vi "Pre Launch Init.vi"(11 "Topic in":refnum<class "Topic.lvclass">) -> (0 "error out":errorcluster, 3 "Topic out":refnum<class "Topic.lvclass">)   [LabVIEW 2017, in "Mediator.lvlib" / "Topic.lvclass"]
doc: "(<B>Filename</B>: Actor Framework.lvlib:Actor.lvclass:Pre Launch Init.vi)\n\nDefines behavior that occurs after the Launch Nested Actor method is invoked but before the actor's Actor Core method begins running.\n\nBy default, this method does nothing. A descendant class may override it to define behavior."
uses:
  Topic.lvclass
  Topic.lvclass/Topic.ctl
  gpm_packages/@cs/event-logger/Source/Composed Log/Log Sink/Log Level.ctl
  gpm_packages/@cs/event-logger/Source/Composed Log/Global Application Log/Message Log Worker.vi
  gpm_packages/@cs/event-logger/Source/Composed Log/Global Application Log/Invalid Reference Error.vi
  gpm_packages/@cs/event-logger/Source/Composed Log/Global Application Log/Get Worker Queue.vi
  gpm_packages/@cs/event-logger/Source/Composed Log/LoggerReference/LoggerReference.lvclass
  <vilib>/ActorFramework/Actor/Actor.lvclass
  gpm_packages/@cs/event-logger/Source/Composed Log/Log Sink/Log Sink.lvclass
  gpm_packages/@cs/event-logger/Source/Composed Log/Composed Log.lvlib
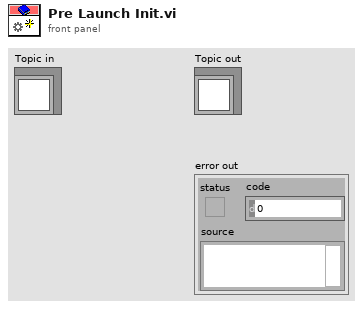
[diagram p1: front panel]
types:
  T1 = typedef "Composed Log.lvlib/Log Sink.lvclass/Log Level.ctl" = enum16{"Debug", "Info", "Warning", "Error", "Critical"}
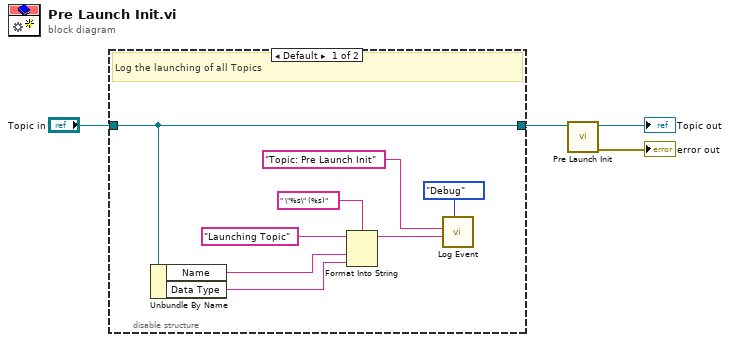
[diagram p0: block diagram]
diagram:
  n1 = disable-structure shown="Default" {
    disable-tunnel: "Topic in" -> [w10 w13]
    disable-tunnel: [w10 w13] -> w1
    frame condition #0 (active) {
      # "Log the launching of all Topics"
      n2 = Unbundle By Name(w10) -> ("Name"=w9:string, "Data Type"=w8:string)
      n3 = Format Into String(format string=" \"%s\" (%s)", initial string="Launching Topic" ("string"), w9, w8) -> (resulting string=w5:string)  [unwired: 1 in, 1 out]
      n4 = call "Log Event.vi"("Event Level"=Log_Level."Debug", "Data To Log"=w5, "SourceID"="Topic: Pre Launch Init") -> ()  [unwired: 7 in, 2 out]
    }
    frame condition #1 {
      # "Remove all logging from this method at compile time"
    }
  }
  n5 = call-parent "Pre Launch Init.vi"("Actor in"=w1) -> ("error out"=→"error out":errorcluster, "Actor out"=→"Topic out":refnum<class "Topic.lvclass">)  [unwired: 9 in]
